vi "Init Logs.vi"(8 "error in (no error)":errorcluster, 9 "Wfm Buffers":refnum<data-value>[](array[refnum]), 10 "Async Data in":T1, 11 "Async Input in":T4={"Device Ref"=18446744073709551615, "Waveforms"=[], "Channels"={"Command Chan Refs"=[], "Command Data Refs"=[], "Command Values"=[], "Status Chan Refs"=[], "Status Data Refs"=[], "Status Values"=[], "System Time"={"System Time"=timestamp(0 s since 1904-01-01), "Data Reference"=0, "Absolute Time Channel Data Ref"=0, "Get Date-Time Channel Data Ref"=0}, "Trigger Chan Refs"=[], "Trigger Data Refs"=[], "Trigger Values"=[]}, "Waveform Logs"=[], "Communication"={"Async Status"=refnum, "Wfm Comm Properties"={"WPL"={"Custom Queue Size"=1, "Use Custom Queue Size?"=FALSE}}, "Shutdown Event"=refnum, "Trigger Event"=refnum, "New File Event"=refnum, "Log Queues"=[], "Async VI Ref"=refnum}, "error"={"status"=FALSE, "code"=0, "source"=""}} {"Device Ref" format="%.0x"; "Channels"."Trigger Data Refs"."Data Reference" format="%.0x"; "Channels"."Trigger Chan Refs" format="%.0x"; "Channels"."System Time"."Get Date-Time Channel Data Ref" format="%.0x"; "Channels"."System Time"."Absolute Time Channel Data Ref" format="%.0x"; "Channels"."System Time"."Channel Data Reference" format="%.0x"; "Channels"."Status Data Refs"."Data Reference" format="%.0x"; "Channels"."Command Data Refs"."Data Reference" format="%.0x"; "Channels"."Status Chan Refs" format="%.0x"; "Channels"."Command Chan Refs" format="%.0x"; "Waveforms"."Waveform Ref in" format="%.0x"; "Waveform Logs"."Node ID" format="%.0x"; "Waveform Logs"."TDMS Error Code"."Data Ref" format="%.0x"; "Waveform Logs"."Missed Samples"."Data Ref" format="%.0x"; "Waveform Logs"."File Status"."Data Ref" format="%.0x"; "Waveform Logs"."Start New File"."Data Ref" format="%.0x"; "Waveform Logs"."Logging Enabled"."Data Ref" format="%.0x"; "Waveform Logs"."Stop Trigger"."Node Data Ref" format="%.0x"; "Waveform Logs"."Stop Trigger"."Node ID" format="%.0x"; "Waveform Logs"."Start Trigger"."Node Data Ref" format="%.0x"; "Waveform Logs"."Start Trigger"."Node ID" format="%.0x"}) -> (0 "error out":errorcluster, 2 "Async Data out":T1, 3 "Async Input out":T4={"Device Ref"=18446744073709551615, "Waveforms"=[], "Channels"={"Command Chan Refs"=[], "Command Data Refs"=[], "Command Values"=[], "Status Chan Refs"=[], "Status Data Refs"=[], "Status Values"=[], "System Time"={"System Time"=timestamp(0 s since 1904-01-01), "Data Reference"=0, "Absolute Time Channel Data Ref"=0, "Get Date-Time Channel Data Ref"=0}, "Trigger Chan Refs"=[], "Trigger Data Refs"=[], "Trigger Values"=[]}, "Waveform Logs"=[], "Communication"={"Async Status"=refnum, "Wfm Comm Properties"={"WPL"={"Custom Queue Size"=1, "Use Custom Queue Size?"=FALSE}}, "Shutdown Event"=refnum, "Trigger Event"=refnum, "New File Event"=refnum, "Log Queues"=[], "Async VI Ref"=refnum}, "error"={"status"=FALSE, "code"=0, "source"=""}} {"Device Ref" format="%.0x"; "Channels"."Trigger Data Refs"."Data Reference" format="%.0x"; "Channels"."Trigger Chan Refs" format="%.0x"; "Channels"."System Time"."Get Date-Time Channel Data Ref" format="%.0x"; "Channels"."System Time"."Absolute Time Channel Data Ref" format="%.0x"; "Channels"."System Time"."Channel Data Reference" format="%.0x"; "Channels"."Status Data Refs"."Data Reference" format="%.0x"; "Channels"."Command Data Refs"."Data Reference" format="%.0x"; "Channels"."Status Chan Refs" format="%.0x"; "Channels"."Command Chan Refs" format="%.0x"; "Waveforms"."Waveform Ref in" format="%.0x"; "Waveform Logs"."Node ID" format="%.0x"; "Waveform Logs"."TDMS Error Code"."Data Ref" format="%.0x"; "Waveform Logs"."Missed Samples"."Data Ref" format="%.0x"; "Waveform Logs"."File Status"."Data Ref" format="%.0x"; "Waveform Logs"."Start New File"."Data Ref" format="%.0x"; "Waveform Logs"."Logging Enabled"."Data Ref" format="%.0x"; "Waveform Logs"."Stop Trigger"."Node Data Ref" format="%.0x"; "Waveform Logs"."Stop Trigger"."Node ID" format="%.0x"; "Waveform Logs"."Start Trigger"."Node Data Ref" format="%.0x"; "Waveform Logs"."Start Trigger"."Node ID" format="%.0x"})   [LabVIEW 2012, in "Waveform Data Logger Engine.lvlib"]
uses:
  Waveform Data Logger Engine.lvlib
  Types/RT Data.ctl
  <vilib>/NI Veristand/Custom Device API/Custom Device Item Ref.ctl
  Types/Inline Waveform Info.ctl
  <vilib>/NI Veristand/Custom Device API/Waveform Data Reference.ctl
  Classes/Waveforms/Waveform Receive/Associated Log.ctl
  <vilib>/NI Veristand/Custom Device API/Custom Device Waveform DataType.ctl
  Types/Channels.ctl
  <vilib>/NI Veristand/Custom Device API/Block Data Reference.ctl
  <vilib>/NI Veristand/Custom Device API/Data Reference.ctl
  Types/System Time.ctl
  Types/Inline Waveform Log Info.ctl
  Shared/Classes/Log File Specifications/Waveform TDMS Log File Specification/Waveform TDMS Log File Specification.lvclass
  Classes/Triggers/Trigger/Trigger.lvclass
  Types/Inline Log Waveform.ctl
  Types/Trigger Settings.ctl
  Types/Log Status.ctl
  Types/Channel.ctl
  Types/Communication.ctl
  Types/Async Status.ctl
  Types/Async State.ctl
  <vilib>/NI Veristand/Custom Device Waveform API/Communication Properties.ctl
  Types/Trigger Event Data.ctl
  Types/Trigger Received.ctl
  Types/New File Event Data.ctl
  Types/Log Queues.ctl
  Types/Async Data.ctl
  <vilib>/NI Veristand/Custom Device Waveform API/Multiple Waveforms Read (DBL)/Multiple Waveforms Read (DBL).lvclass
  Classes/Waveforms/Utilities/Reference Dictionary/Reference Dictionary.lvclass
  Types/Wfm Acq Data.ctl
  Classes/Waveforms/Waveform Receive/Waveform Receive.lvclass
  Classes/Waveforms/Waveform Log/Waveform Log.lvclass
  Types/Async Communication.ctl
  Types/Check File Loop Cmd.ctl
  Classes/Waveforms/Buffer/Waveform Buffer/Waveform Buffer.lvclass
  Classes/Waveforms/Waveform Log/Log Waveform.ctl
  Classes/Waveforms/Waveform Log/Waveform Information.ctl
  Classes/Waveforms/Waveform Log/Waveform Data Type.ctl
  <vilib>/NI VeriStand/Custom Device API/Custom Device API.lvlib
  <vilib>/NI VeriStand/Custom Device Waveform API/NI_VS Custom Device Waveform API.lvlib
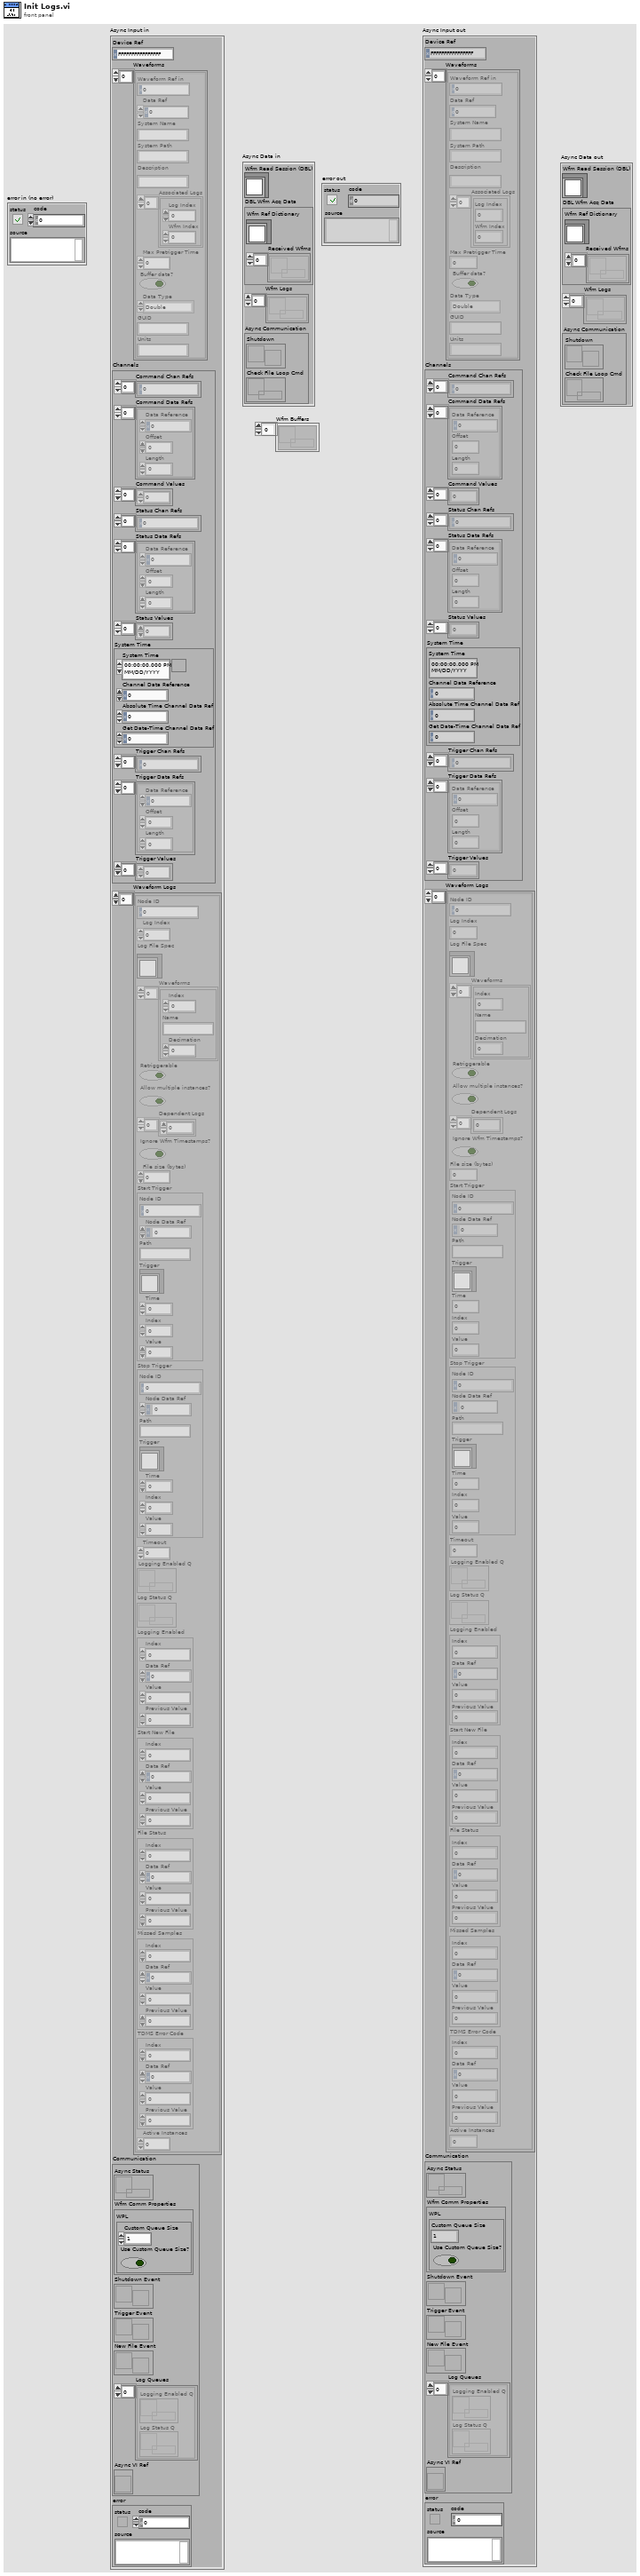
[diagram p1: front panel]
types:
  T1 = typedef "Waveform Data Logger Engine.lvlib/Async Data.ctl" = cluster{"Wfm Read Session (DBL)":refnum<class "Multiple Waveforms Read (DBL).lvclass">, "DBL Wfm Acq Data":T2, "Wfm Logs":refnum<data-value>[], "Async Communication":T3}
  T2 = typedef "Waveform Data Logger Engine.lvlib/Wfm Acq Data.ctl" = cluster{"Wfm Ref Dictionary":refnum<class "Reference Dictionary.lvclass">, "Received Wfms":refnum<data-value>[]}
  T3 = typedef "Waveform Data Logger Engine.lvlib/Async Communication.ctl" = cluster{"Shutdown":refnum<user-event>, "Check File Loop Cmd":refnum<queue>}
  T4 = typedef "Waveform Data Logger Engine.lvlib/RT Data.ctl" = cluster{"Device Ref":T5, "Waveforms":T6[], "Channels":T10, "Waveform Logs":T14[], "Communication":T18, "error":errorcluster}
  T5 = typedef "Custom Device API.lvlib/Custom Device Item Ref.ctl" = u64
  T6 = typedef "Waveform Data Logger Engine.lvlib/Inline Waveform Info.ctl" = cluster{"Waveform Ref in":T5, "Data Ref":T7, "System Name":string, "System Path":string, "Description":string, "Associated Logs":T8[], "Max Pretrigger Time":dbl, "Buffer data?":bool, "Data Type":T9, "GUID":string, "Units":string}
  T7 = typedef "Custom Device API.lvlib/Waveform Data Reference.ctl" = i32
  T8 = typedef "Waveform Data Logger Engine.lvlib/Waveform Receive.lvclass/Associated Log.ctl" = cluster{"Log Index":i32, "Wfm Index":i32}
  T9 = typedef "Custom Device API.lvlib/Custom Device Waveform DataType.ctl" = enum16{"Double", "Complex Double"}
  T10 = typedef "Waveform Data Logger Engine.lvlib/Channels.ctl" = cluster{"Command Chan Refs":T5[], "Command Data Refs":T11[], "Command Values":dbl[], "Status Chan Refs":T5[], "Status Data Refs":T11[], "Status Values":dbl[], "System Time":T13, "Trigger Chan Refs":T5[], "Trigger Data Refs":T11[], "Trigger Values":dbl[]}
  T11 = typedef "Custom Device API.lvlib/Block Data Reference.ctl" = cluster{"Data Reference":T12, "Offset":i32, "Length":i32}
  T12 = typedef "Custom Device API.lvlib/Data Reference.ctl" = i32
  T13 = typedef "Waveform Data Logger Engine.lvlib/System Time.ctl" = cluster{"System Time":timestamp, "Data Reference":T12, "Absolute Time Channel Data Ref":T12, "Get Date-Time Channel Data Ref":T12}
  T14 = typedef "Waveform Data Logger Engine.lvlib/Inline Waveform Log Info.ctl" = cluster{"Node ID":T5, "Log Index":i32, "Log File Spec":refnum<class "Waveform TDMS Log File Specification.lvclass">, "Waveforms":T15[], "Retriggerable":bool, "Allow multiple instances?":bool, "Dependent Logs":i32[], "Ignore Wfm Timestamps?":bool, "File size (bytes)":i64, "Start Trigger":T16, "Stop Trigger":T16, "Timeout":dbl, "Logging Enabled Q":refnum<queue>, "Log Status Q":refnum<queue>, "Logging Enabled":T17, "Start New File":T17, "File Status":T17, "Missed Samples":T17, "TDMS Error Code":T17, "Active Instances":i32}
  T15 = typedef "Waveform Data Logger Engine.lvlib/Inline Log Waveform.ctl" = cluster{"Index":i32, "Name":string, "Decimation":u32}
  T16 = typedef "Waveform Data Logger Engine.lvlib/Trigger Settings.ctl" = cluster{"Node ID":T5, "Node Data Ref":i32, "Path":string, "Trigger":refnum<class "Trigger.lvclass">, "Time":dbl, "Index":i32, "Value":dbl}
  T17 = typedef "Waveform Data Logger Engine.lvlib/Channel.ctl" = cluster{"Index":i32, "Data Ref":T12, "Value":dbl, "Previous Value":dbl}
  T18 = typedef "Waveform Data Logger Engine.lvlib/Communication.ctl" = cluster{"Async Status":refnum<queue>, "Wfm Comm Properties":T19, "Shutdown Event":refnum<user-event>, "Trigger Event":refnum<user-event>, "New File Event":refnum<user-event>, "Log Queues":T20[], "Async VI Ref":refnum<vi>}
  T19 = typedef "NI_VS Custom Device Waveform API.lvlib/Communication Properties.ctl" = cluster{"WPL":cluster{"Custom Queue Size":i32, "Use Custom Queue Size?":bool}}
  T20 = typedef "Waveform Data Logger Engine.lvlib/Log Queues.ctl" = cluster{"Logging Enabled Q":refnum<queue>, "Log Status Q":refnum<queue>}
  T21 = typedef "Waveform Data Logger Engine.lvlib/Waveform Log.lvclass/Waveform Data Type.ctl" = enum16{"Double", "ComplexDouble"}
  T22 = typedef "Waveform Data Logger Engine.lvlib/Waveform Log.lvclass/Log Waveform.ctl" = cluster{"Buffer Ref":refnum<data-value>, "Wfm Info":T23}
  T23 = typedef "Waveform Data Logger Engine.lvlib/Waveform Log.lvclass/Waveform Information.ctl" = cluster{"Name":string, "Wfm Data Type":T21, "Decimation":u32}
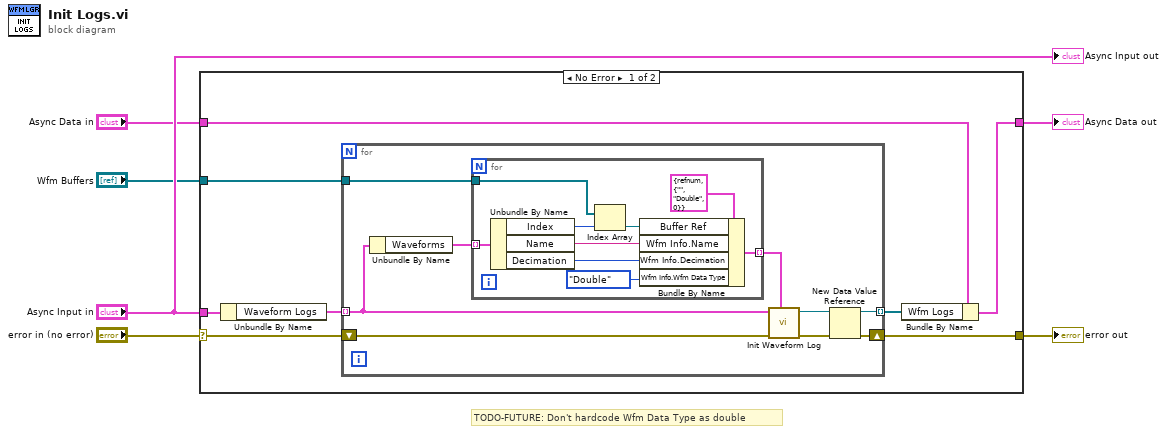
[diagram p0: block diagram]
diagram:
  # "TODO-FUTURE: Don't hardcode Wfm Data Type as double"
  n1 = case shown="No Error" "error in (no error)" {
    selector: "error in (no error)" -> [w8 w34]
    tunnel: [w9 w34] -> w5
    tunnel: "Async Data in" -> [w14 w33]
    tunnel: [w13 w33] -> w4
    tunnel: "Async Input in" -> [w12 _]
    tunnel: "Wfm Buffers" -> [w7 _]
    frame No Error {
      n2 = Unbundle By Name(w12) -> ("Waveform Logs"=w11:T14[])
      n3 = for {
        tunnel: w11 -> [w18] mode=indexing
        shift-right: [w21] -> w9
        shift-left: w8 -> [w19]
        tunnel: [w20] -> w10 mode=indexing
        tunnel: w7 -> [w16]
        n4 = Unbundle By Name(w18) -> ("Waveforms"=w17:T15[])
        n5 = for {
          tunnel: w17 -> [w32] mode=indexing
          tunnel: w16 -> [w31]
          tunnel: [w26] -> w15 mode=indexing
          n6 = Unbundle By Name(w32) -> ("Index"=w28:i32, "Name"=w27:string, "Decimation"=w25:u32)
          n7 = Index Array(array=w31, index=w28) -> (element=w29:refnum<data-value>)
          n8 = Bundle By Name(cluster=T22 {"Buffer Ref"=refnum, "Wfm Info"={"Name"="", "Wfm Data Type"=enum."Double", "Decimation"=0}} ("Log Waveform"), "Buffer Ref"=w29, "Wfm Info.Name"=w27, "Wfm Info.Decimation"=w25, "Wfm Info.Wfm Data Type"=Waveform_Data_Type."Double") -> (w26:T22)
        }
        n9 = call "Init Waveform Log.vi"("Waveforms"=w15, "error in (no error)"=w19, "Waveform Log Info"=w18) -> ("error out"=w22:errorcluster, "Waveform Log out"=w23:refnum<class "Waveform Log.lvclass">)  [unwired: 7 in]
        n10 = New Data Value Reference(data value=w23, error in=w22) -> (data value reference=w20:refnum<data-value>, error out=w21:errorcluster)
      }
      n11 = Bundle By Name(cluster=w14, "Wfm Logs"=w10) -> (w13:T1)
    }
    frame Error {
    }
  }
  "Async Data out" <- w4
  "error out" <- w5
  "Async Input out" <- "Async Input in"
